vi "Connect.vi"(8 "error in":errorcluster, 10 "Additional Information":string, 11 "DB-Engine in":refnum<class "DB-Interface.lvclass">) -> (0 "error out":errorcluster, 3 "DB-Engine out":refnum<class "DB-Interface.lvclass">)   [LabVIEW 2014, in "hse-db.lvlib" / "DB-Interface.lvclass"]
doc: "Connect.\n\n-- This method is just a prototype --"
uses:
  DB-Interface.lvclass
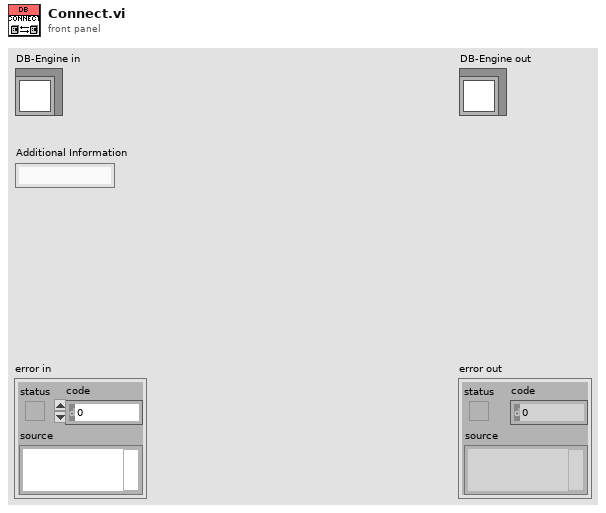
[diagram p1: front panel]
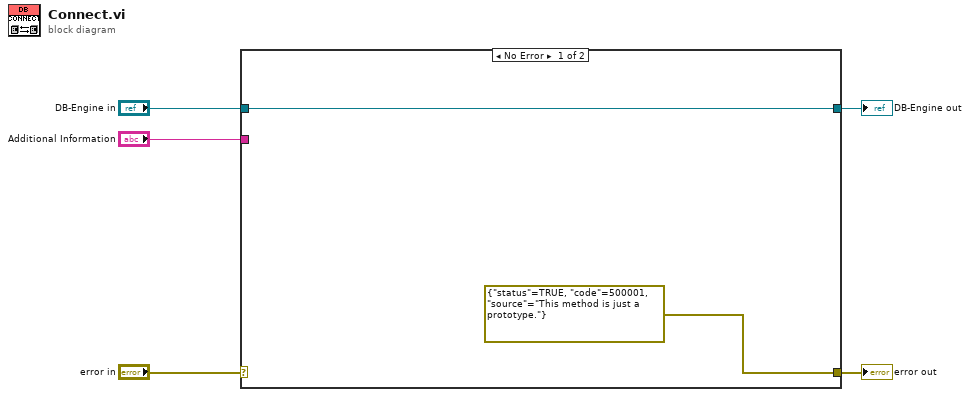
[diagram p0: block diagram]
diagram:
  n1 = case shown="No Error" "error in" {
    selector: "error in" -> [_ w9]
    tunnel: [errorcluster {"status"=TRUE, "code"=500001, "source"="This method is just a prototype."} ("error IO") w9] -> w4
    tunnel: [w7 w8] -> w2
    tunnel: "DB-Engine in" -> [w7 w8]
    tunnel: "Additional Information" -> [_ _]
    frame No Error {
    }
    frame Error {
    }
  }
  "error out" <- w4
  "DB-Engine out" <- w2
